vi "TRI.vi"(0 "System no.":i32=1 min=1 max=4 step=1, 2 "TriggerIn to command":string[](array[string]), 3 "Trigger status":bool[](array[boolean]), 5 "error in":errorcluster) -> (19 "error out":errorcluster)   [LabVIEW 2020]
doc: "Enables or disables the Trigger Input mode which was set with CTI. TRI has no effect on DIO?, i.e. DIO? will always answer the current logical state of the input line level even if TRI is enabled.\n\nC-709: Check controller user manual for available input trigger numbers."
panel:
  # "Enables or disables the TRrigger Input mode which was set with CTI."
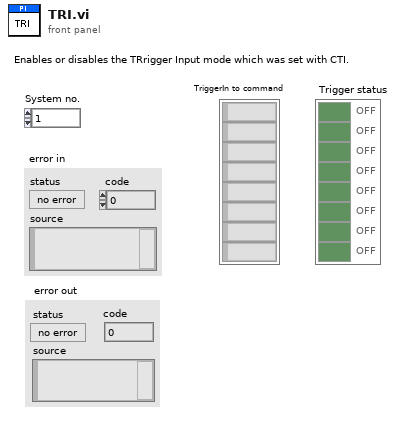
[diagram p1: front panel]
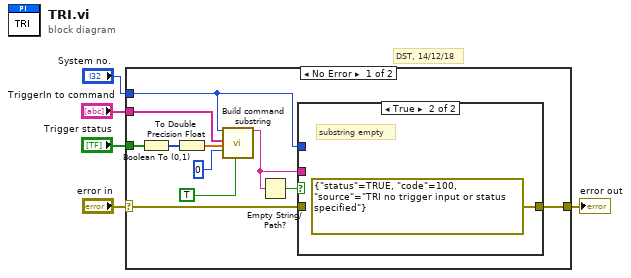
[diagram p0: block diagram]
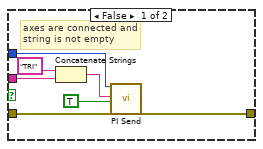
[diagram p2: hidden frame]
diagram:
  # "DST, 14/12/18"
  n1 = case shown="No Error" "error in" {
    selector: "error in" -> [w8 w25]
    tunnel: [w16 w25] -> w5
    tunnel: "System no." -> [w11 _]
    tunnel: "TriggerIn to command" -> [w15 _]
    tunnel: "Trigger status" -> [w14 _]
    frame No Error {
      n2 = Boolean To (0,1)(Boolean=w14) -> (0, 1=w13:i16[])
      n3 = To Double Precision Float(number=w13) -> (double precision float=w12:dbl[])
      n4 = call "Build command substring.vi"("System no."=w11, "Affected axes"=w15, "Parameters"=w12, "No. of digits"=i16 0 ("No.of digits"), "With space?"=TRUE) -> ("Command substring"=w7:string)  [unwired: 2 in, 12 out]
      n5 = Empty String/Path?(string/path=w7) -> (empty?=w6:bool)
      n6 = case shown="True" w6 {
        tunnel: w7 -> [w22 _]
        tunnel: [w18 errorcluster {"status"=TRUE, "code"=100, "source"="TRI no trigger input or status specified"} ("error out")] -> w16
        tunnel: w8 -> [w19 _]
        tunnel: w11 -> [w17 _]
        frame False {
          # "axes are connected and\nstring is not empty"
          n7 = Concatenate Strings("TRI", w22) -> (w20:string)
          n8 = call "PI Send.vi"("System no."=w17, "String to send"=w20, "Attach termination char.?"=TRUE ("Attach Linefeed?"), "error in"=w19) -> ("error out"=w18:errorcluster)  [unwired: 2 in, 13 out]
        }
        frame True {
          # "substring empty"
        }
      }
    }
    frame Error {
    }
  }
  "error out" <- w5
